vi "Memory Cell to int.vi"(7 "Field Selector":T1, 10 "Memory Cell":T2) -> (2 "Int out":i32)   [LabVIEW 2017]
uses:
  Type Definitions/Memory Cell.ctl
  Type Definitions/Memory Cell Type Enum.ctl
  Type Definitions/Cell Selector.ctl
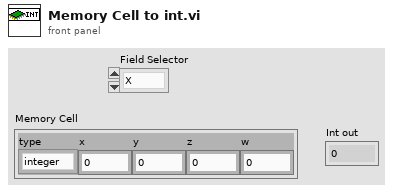
[diagram p1: front panel]
types:
  T1 = typedef "Cell Selector.ctl" = enum16{"X", "Y", "Z", "W"}
  T2 = typedef "Memory Cell.ctl" = cluster{"type":T3, "x":dbl, "y":dbl, "z":dbl, "w":dbl}
  T3 = typedef "Memory Cell Type Enum.ctl" = enum16{"integer", "float", "vector", "rotation"}
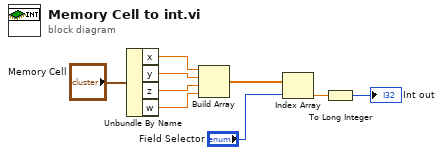
[diagram p0: block diagram]
diagram:
  n1 = Unbundle By Name("Memory Cell") -> ("x"=w8:dbl, "y"=w7:dbl, "z"=w6:dbl, "w"=w5:dbl)
  n2 = Build Array(w8, w7, w6, w5) -> (w4:dbl[])
  n3 = Index Array(array=w4, index="Field Selector") -> (element=w1:dbl)
  n4 = To Long Integer(number=w1) -> (32bit integer=→"Int out":i32)
